vi "Parse Record.vi"(11 "record":T3 {"type" format="%04x"; "timestamp" format="%08x"; "msgact" format="%04x"; "data" format="%08x"; "timestamph" format="%08x"}) -> (0 "specific errors":T2, 1 "time stamp":dbl, 2 "valid":bool, 3 "data word":u32 format="%032b", 5 "message info":T1)   [LabVIEW 2020, in "Ballard ARINC 429 Engine.lvlib" / "Custom Device.lvlib"]
uses:
  Custom Device.lvlib
  <instrlib>/BTICardLib/Public/Controls/429 Record.ctl
  <instrlib>/BTICardLib/BTICardLV.lvlib
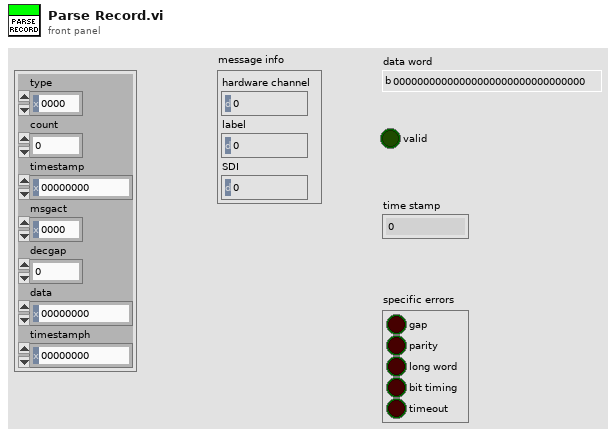
[diagram p1: front panel]
types:
  T1 = cluster{"hardware channel":u8, "label":u8, "SDI":u8}
  T2 = cluster{"gap":bool, "parity":bool, "long word":bool, "bit timing":bool, "timeout":bool}
  T3 = typedef "BTICardLV.lvlib/429 Record.ctl" = cluster{"type":u16, "count":u16, "timestamp":u32, "msgact":u16, "decgap":u16, "data":u32, "timestamph":u32}
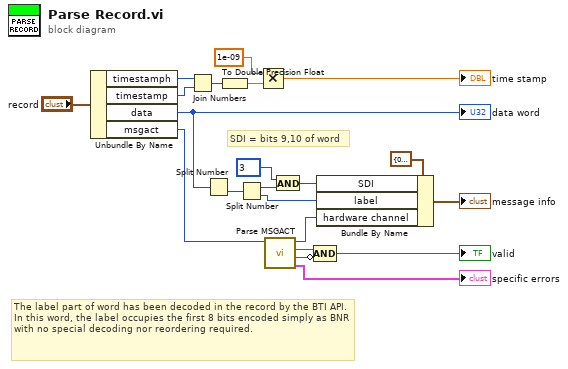
[diagram p0: block diagram]
diagram:
  # "SDI = bits 9,10 of word"
  # "The label part of word has been decoded in the record by the BTI API. In this word, the label occupies the first 8 bits encoded simply as BNR with no special decoding nor reordering required."
  n1 = Unbundle By Name("record") -> ("timestamph"=w12:u32, "timestamp"=w11:u32, "data"=w2:u32, "msgact"=w20:u16)
  "data word" <- w2
  n2 = Join Numbers(hi=w12, lo=w11) -> ((hi.lo)=w13:u64)
  n3 = Split Number(x=w2) -> (lo(x)=w7:u16)  [unwired: 1 out]
  n4 = To Double Precision Float(number=w13) -> (double precision float=w15:dbl)
  n5 = Split Number(x=w7) -> (hi(x)=w8:u8, lo(x)=w1:u8)
  n6 = Multiply(x=1e-09 ("y"), y=w15) -> (x*y=→"time stamp":dbl)
  n7 = call "Parse MSGACT.vi"("msgact"=w20) -> ("specific errors"=→"specific errors":T2, "receiving error"=w17:bool, "hit"=w18:bool, "hardware channel"=w3:u8)  [unwired: 7 in]
  n8 = And(x=u8 3, y=w8) -> (x .and. y?=w4:u8)
  n9 = Compound Arithmetic op=AND(w18, invert w17) -> (→"valid":bool)
  n10 = Bundle By Name(cluster=T1 {"hardware channel"=0, "label"=0, "SDI"=0} ("message info"), "SDI"=w4, "label"=w1, "hardware channel"=w3) -> (→"message info":T1)
